vi "subbocht.vi"(4 "tijdsinterval 6":dbl, 5 "Boolean":bool, 6 "tijdsinterval 8":dbl, 7 "tijdsinterval in":dbl, 8 "tijdsinterval 7":dbl, 9 "tijdsinterval 5":dbl, 10 "tijdsinterval 4":dbl, 11 "tijdsinterval 3":dbl) -> ()   [LabVIEW 2019]
uses:
  Global 1.vi
  <vilib>/myRIO/Common/Instrument Driver Framework/Utilities/typedefs/Analog Scaling Constants.ctl
  <vilib>/myRIO/Common/Instrument Driver Framework/Utilities/typedefs/Analog Scaling Constants List.ctl
  <vilib>/myRIO/Common/Instrument Driver Framework/myRIO v1.0/AO/typedefs/AO Channels Enum.ctl
  <vilib>/myRIO/Common/Instrument Driver Framework/myRIO v1.0/AO/typedefs/AO Channels List.ctl
  <vilib>/myRIO/Common/Instrument Driver Framework/Utilities/typedefs/Generic FPGA Reference.ctl
  <vilib>/myRIO/Common/Instrument Driver Framework/Utilities/typedefs/myRIO v1.0 Reference.ctl
  <vilib>/myRIO/Common/Instrument Driver Framework/Utilities/typedefs/Hardware Version Enum.ctl
  <vilib>/myRIO/Common/Instrument Driver Framework/Utilities/typedefs/myRIO Generic Hardware Reference.ctl
  <vilib>/myRIO/Instrument Drivers/Onboard IO/AO/typedefs/AO Reference.ctl
  <vilib>/myRIO/Instrument Drivers/Onboard IO/AO/AO.lvlib
  <vilib>/myRIO/Instrument Drivers/Onboard IO/AO/vis/Write.vi
  <vilib>/userDefined/High Color/nirio_resource_hc.ctl
  <vilib>/myRIO/Common/Instrument Driver Framework/myRIO v1.0/AO/vis/myRIO v1.1 Open AO.vi
  <vilib>/myRIO/Instrument Drivers/Onboard IO/AO/vis/myRIO AO Open.xnode
  <vilib>/myRIO/Common/Instrument Driver Framework/Utilities/vis/Is FPGA Ref Available.vi
  <vilib>/myRIO/Express VI/Onboard IO/AO/AO Express VI.xnode
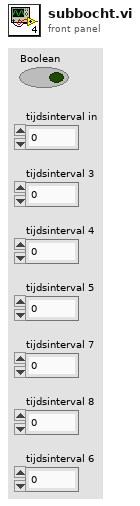
[diagram p1: front panel]
types:
  T1 = typedef "AO.lvlib/AO Reference.ctl" = cluster{"myRIO Reference":T2, "AO Channel List":T6, "AO Scaling Constant List":T8}
  T2 = typedef "myRIO Generic Hardware Reference.ctl" = cluster{"myRIO Model":T3, "myRIO Hardware Reference":T4}
  T3 = typedef "Hardware Version Enum.ctl" = enum16{"Unknown", "myRIO-1900", "myRIO-1950", "roboRIO", "NI ELVIS RIO CM", "ELVIS III"}
  T4 = typedef "myRIO v1.0 Reference.ctl" = cluster{"Generic FPGA Reference":T5, "Allow multiple opens":bool}
  T5 = typedef "Generic FPGA Reference.ctl" = refnum<k20>
  T6 = typedef "AO Channels List.ctl" = T7[]
  T7 = typedef "AO Channels Enum.ctl" = enum16{"Not Connected", "AudioOut/Left", "AudioOut/Right", "C/AO0", "C/AO1", "A/AO0", "A/AO1", "B/AO0", "B/AO1"}
  T8 = typedef "Analog Scaling Constants List.ctl" = T9[]
  T9 = typedef "Analog Scaling Constants.ctl" = cluster{"LSB Weight (Volts)":dbl, "Offset (Volts)":dbl, "Signed?":bool}
  T10 = typedef "nirio_resource_hc.ctl" = tag
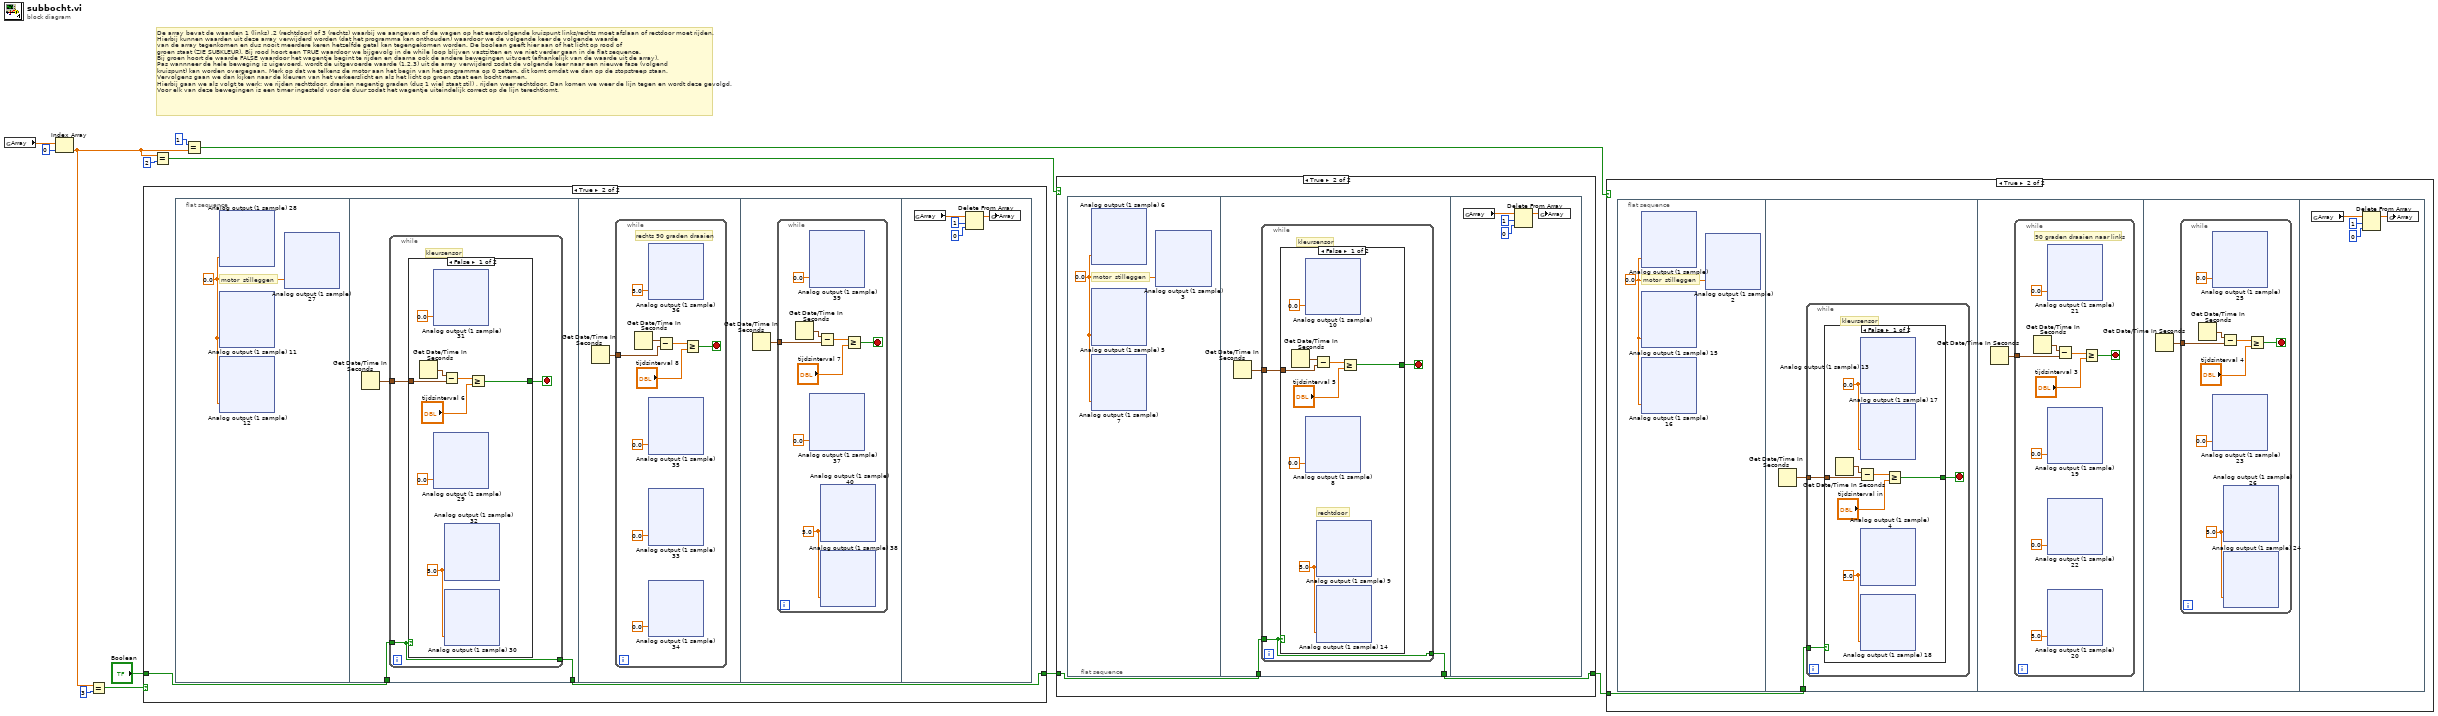
[diagram p0: block diagram]
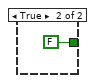
[diagram p3: hidden frame]
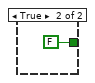
[diagram p5: hidden frame]
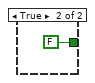
[diagram p7: hidden frame]
diagram:
  # "De array bevat de waarden 1 (links) ,2 (rechtdoor) of 3 (rechts) waarbij we aangeven of de wagen op het eerstvolgende kruispunt links/rechts moet afslaan of rectdoor moet rijden.\nHierbij kunnen waarden uit deze array verwijderd worden (dat het programma kan onthouden) waardoor we de volgende keer de volgende waarde \nvan de array tegenkomen en dus nooit meerdere keren hetzelfde getal kan tegengekomen worden. De boolean geeft hier aan of het licht op rood of \ngroen staat (ZIE SUBKLEUR). Bij rood hoort een TRUE waardoor we bijgevolg in de while loop blijven vastzitten en we niet verder gaan in de flat sequence.\nBij groen hoort de waarde FALSE waardoor het wagentje begint te rijden en daarna ook de andere bewegingen uitvoert (afhankelijk van de waarde uit de array).\nPas wannneer de hele beweging is uigevoerd, wordt de uitgevoerde waarde (1,2,3) uit de array verwijderd zodat de volgende keer naar een nieuwe fase (volgend\nkruispunt) kan worden overgegaan. Merk op dat we telkens de motor aan het begin van het programma op 0 zetten, dit komt omdat we dan op de stopstreep staan.\nVervolgens gaan we dan kijken naar de kleuren van het verkeerslicht en als het licht op groen staat een bocht nemen.\nHierbij gaan we als volgt te werk: we rijden rechttdoor, draaien negentig graden (dus 1 wiel staat stil) , rijden weer rechtdoor. Dan komen we weer de lijn tegen en wordt deze gevolgd.\nVoor elk van deze bewegingen is een timer ingesteld voor de duur zodat het wagentje uiteindelijk correct op de lijn terechtkomt."
  n1 = global read "Global 1.vi" "Array"() -> (w4:dbl[])
  n2 = Index Array(array=w4, index=0) -> (element=w6:dbl)
  n3 = Equal?(x=w6, y=3) -> (x = y?=w3:bool)
  n4 = case shown="True" w3 {
    tunnel: "Boolean" -> [w13 w15]
    tunnel: [w13 w14] -> w11
    frame False {
    }
    frame True {
      n5 = flat-sequence {
        tunnel: w15 -> [w167]
        tunnel: [w166] -> w14
        frame #0 {
          w16 = 0.0
          # "motor  stilleggen"
          n6 = xnode "Analog output (1 sample) 28"("A/AO1 (Pin 4)"=w16) -> ()  [unwired: 1 in, 1 out]
          n7 = xnode "Analog output (1 sample) 11"("B/AO0 (Pin 2)"=w16) -> ()  [unwired: 1 in, 1 out]
          n8 = xnode "Analog output (1 sample) 12"("A/AO0 (Pin 2)"=w16) -> ()  [unwired: 1 in, 1 out]
          n9 = xnode "Analog output (1 sample) 27"("B/AO1 (Pin 4)"=w16) -> ()  [unwired: 1 in, 1 out]
        }
        frame #1 {
          n10 = Get Date/Time In Seconds() -> (seconds since 1Jan1904=w165:timestamp)
          n11 = while {
            tunnel: w167 -> [w169]
            tunnel: [w169] -> w166
            tunnel: w165 -> [w168]
            stop <- w170 stop-if-true
            # "kleursensor"
            n12 = case shown="False" w169 {
              tunnel: [w171 FALSE] -> w170
              tunnel: w168 -> [w172 _]
              frame False {
                w177 = 5.0
                n13 = Get Date/Time In Seconds() -> (seconds since 1Jan1904=w173:timestamp)
                n14 = xnode "Analog output (1 sample) 31"("A/AO1 (Pin 4)"=0.0) -> ()  [unwired: 1 in, 1 out]
                n15 = xnode "Analog output (1 sample) 29"("B/AO1 (Pin 4)"=0.0) -> ()  [unwired: 1 in, 1 out]
                n16 = Subtract(x=w173, y=w172) -> (x-y=w175:dbl)
                n17 = xnode "Analog output (1 sample) 32"("A/AO0 (Pin 2)"=w177) -> ()  [unwired: 1 in, 1 out]
                n18 = xnode "Analog output (1 sample) 30"("B/AO0 (Pin 2)"=w177) -> ()  [unwired: 1 in, 1 out]
                n19 = Greater Or Equal?(x=w175, y="tijdsinterval 6") -> (x >= y?=w171:bool)
              }
              frame True {
              }
            }
          }
        }
        frame #2 {
          n20 = Get Date/Time In Seconds() -> (seconds since 1Jan1904=w328:timestamp)
          n21 = while {
            tunnel: w328 -> [w330]
            stop <- w331 stop-if-true
            # "rechts 90 graden draaien"
            n22 = Get Date/Time In Seconds() -> (seconds since 1Jan1904=w334:timestamp)
            n23 = xnode "Analog output (1 sample) 36"("A/AO0 (Pin 2)"=5.0) -> ()  [unwired: 1 in, 1 out]
            n24 = xnode "Analog output (1 sample) 35"("A/AO1 (Pin 4)"=0.0) -> ()  [unwired: 1 in, 1 out]
            n25 = xnode "Analog output (1 sample) 33"("B/AO1 (Pin 4)"=0.0) -> ()  [unwired: 1 in, 1 out]
            n26 = xnode "Analog output (1 sample) 34"("B/AO0 (Pin 2)"=0.0) -> ()  [unwired: 1 in, 1 out]
            n27 = Subtract(x=w334, y=w330) -> (x-y=w332:dbl)
            n28 = Greater Or Equal?(x=w332, y="tijdsinterval 8") -> (x >= y?=w331:bool)
          }
        }
        frame #3 {
          n29 = Get Date/Time In Seconds() -> (seconds since 1Jan1904=w486:timestamp)
          n30 = while {
            tunnel: w486 -> [w488]
            stop <- w487 stop-if-true
            w493 = 5.0
            n31 = Get Date/Time In Seconds() -> (seconds since 1Jan1904=w491:timestamp)
            n32 = xnode "Analog output (1 sample) 39"("A/AO1 (Pin 4)"=0.0) -> ()  [unwired: 1 in, 1 out]
            n33 = xnode "Analog output (1 sample) 37"("B/AO1 (Pin 4)"=0.0) -> ()  [unwired: 1 in, 1 out]
            n34 = Subtract(x=w491, y=w488) -> (x-y=w489:dbl)
            n35 = xnode "Analog output (1 sample) 40"("A/AO0 (Pin 2)"=w493) -> ()  [unwired: 1 in, 1 out]
            n36 = xnode "Analog output (1 sample) 38"("B/AO0 (Pin 2)"=w493) -> ()  [unwired: 1 in, 1 out]
            n37 = Greater Or Equal?(x=w489, y="tijdsinterval 7") -> (x >= y?=w487:bool)
          }
        }
        frame #4 {
          n38 = global read "Global 1.vi" "Array"() -> (w645:dbl[])
          n39 = Delete From Array(array=w645, length=1, index=0) -> (array with subset deleted=w646:dbl[])  [unwired: 1 out]
          n40 = global write "Global 1.vi" "Array"(w646) -> ()
        }
      }
    }
  }
  n41 = Equal?(x=w6, y=2) -> (x = y?=w2:bool)
  n42 = Equal?(x=1, y=w6) -> (x = y?=w1:bool)
  n43 = case shown="True" w2 {
    tunnel: w11 -> [w647 w649]
    tunnel: [w647 w648] -> w12
    frame False {
    }
    frame True {
      n44 = flat-sequence {
        tunnel: w649 -> [w801]
        tunnel: [w800] -> w648
        frame #0 {
          w650 = 0.0
          # "motor  stilleggen"
          n45 = xnode "Analog output (1 sample) 6"("A/AO1 (Pin 4)"=w650) -> ()  [unwired: 1 in, 1 out]
          n46 = xnode "Analog output (1 sample) 5"("B/AO0 (Pin 2)"=w650) -> ()  [unwired: 1 in, 1 out]
          n47 = xnode "Analog output (1 sample) 7"("A/AO0 (Pin 2)"=w650) -> ()  [unwired: 1 in, 1 out]
          n48 = xnode "Analog output (1 sample) 3"("B/AO1 (Pin 4)"=w650) -> ()  [unwired: 1 in, 1 out]
        }
        frame #1 {
          n49 = Get Date/Time In Seconds() -> (seconds since 1Jan1904=w799:timestamp)
          n50 = while {
            tunnel: w801 -> [w803]
            tunnel: [w803] -> w800
            tunnel: w799 -> [w802]
            stop <- w804 stop-if-true
            # "kleursensor"
            n51 = case shown="False" w803 {
              tunnel: [w805 FALSE] -> w804
              tunnel: w802 -> [w806 _]
              frame False {
                w811 = 5.0
                # "rechtdoor"
                n52 = Get Date/Time In Seconds() -> (seconds since 1Jan1904=w809:timestamp)
                n53 = xnode "Analog output (1 sample) 10"("A/AO1 (Pin 4)"=0.0) -> ()  [unwired: 1 in, 1 out]
                n54 = xnode "Analog output (1 sample) 8"("B/AO1 (Pin 4)"=0.0) -> ()  [unwired: 1 in, 1 out]
                n55 = Subtract(x=w809, y=w806) -> (x-y=w807:dbl)
                n56 = xnode "Analog output (1 sample) 9"("A/AO0 (Pin 2)"=w811) -> ()  [unwired: 1 in, 1 out]
                n57 = xnode "Analog output (1 sample) 14"("B/AO0 (Pin 2)"=w811) -> ()  [unwired: 1 in, 1 out]
                n58 = Greater Or Equal?(x=w807, y="tijdsinterval 5") -> (x >= y?=w805:bool)
              }
              frame True {
              }
            }
          }
        }
        frame #2 {
          n59 = global read "Global 1.vi" "Array"() -> (w964:dbl[])
          n60 = Delete From Array(array=w964, length=1, index=0) -> (array with subset deleted=w965:dbl[])  [unwired: 1 out]
          n61 = global write "Global 1.vi" "Array"(w965) -> ()
        }
      }
    }
  }
  n62 = case shown="True" w1 {
    tunnel: w12 -> [_ w966]
    frame False {
    }
    frame True {
      n63 = flat-sequence {
        tunnel: w966 -> [w1117]
        frame #0 {
          w967 = 0.0
          # "motor  stilleggen"
          n64 = xnode "Analog output (1 sample)"("A/AO1 (Pin 4)"=w967) -> ()  [unwired: 1 in, 1 out]
          n65 = xnode "Analog output (1 sample) 15"("B/AO1 (Pin 4)"=w967) -> ()  [unwired: 1 in, 1 out]
          n66 = xnode "Analog output (1 sample) 16"("A/AO0 (Pin 2)"=w967) -> ()  [unwired: 1 in, 1 out]
          n67 = xnode "Analog output (1 sample) 2"("B/AO0 (Pin 2)"=w967) -> ()  [unwired: 1 in, 1 out]
        }
        frame #1 {
          n68 = Get Date/Time In Seconds() -> (seconds since 1Jan1904=w1116:timestamp)
          n69 = while {
            tunnel: w1117 -> [w1119]
            tunnel: w1116 -> [w1118]
            stop <- w1120 stop-if-true
            # "kleursensor"
            n70 = case shown="False" w1119 {
              tunnel: [w1122 FALSE] -> w1120
              tunnel: w1118 -> [w1121 _]
              frame False {
                w1126 = 0.0
                w1127 = 5.0
                n71 = Get Date/Time In Seconds() -> (seconds since 1Jan1904=w1125:timestamp)
                n72 = Subtract(x=w1125, y=w1121) -> (x-y=w1123:dbl)
                n73 = xnode "Analog output (1 sample) 13"("A/AO1 (Pin 4)"=w1126) -> ()  [unwired: 1 in, 1 out]
                n74 = xnode "Analog output (1 sample) 17"("B/AO1 (Pin 4)"=w1126) -> ()  [unwired: 1 in, 1 out]
                n75 = xnode "Analog output (1 sample) 4"("A/AO0 (Pin 2)"=w1127) -> ()  [unwired: 1 in, 1 out]
                n76 = xnode "Analog output (1 sample) 18"("B/AO0 (Pin 2)"=w1127) -> ()  [unwired: 1 in, 1 out]
                n77 = Greater Or Equal?(x=w1123, y="tijdsinterval in") -> (x >= y?=w1122:bool)
              }
              frame True {
              }
            }
          }
        }
        frame #2 {
          n78 = Get Date/Time In Seconds() -> (seconds since 1Jan1904=w1277:timestamp)
          n79 = while {
            tunnel: w1277 -> [w1280]
            stop <- w1279 stop-if-true
            # "90 graden draaien naar links"
            n80 = Get Date/Time In Seconds() -> (seconds since 1Jan1904=w1283:timestamp)
            n81 = xnode "Analog output (1 sample) 21"("A/AO1 (Pin 4)"=0.0) -> ()  [unwired: 1 in, 1 out]
            n82 = xnode "Analog output (1 sample) 19"("B/AO1 (Pin 4)"=0.0) -> ()  [unwired: 1 in, 1 out]
            n83 = xnode "Analog output (1 sample) 22"("A/AO0 (Pin 2)"=0.0) -> ()  [unwired: 1 in, 1 out]
            n84 = xnode "Analog output (1 sample) 20"("B/AO0 (Pin 2)"=5.0) -> ()  [unwired: 1 in, 1 out]
            n85 = Subtract(x=w1283, y=w1280) -> (x-y=w1281:dbl)
            n86 = Greater Or Equal?(x=w1281, y="tijdsinterval 3") -> (x >= y?=w1279:bool)
          }
        }
        frame #3 {
          n87 = Get Date/Time In Seconds() -> (seconds since 1Jan1904=w1435:timestamp)
          n88 = while {
            tunnel: w1435 -> [w1437]
            stop <- w1436 stop-if-true
            w1442 = 5.0
            n89 = Get Date/Time In Seconds() -> (seconds since 1Jan1904=w1440:timestamp)
            n90 = xnode "Analog output (1 sample) 25"("A/AO1 (Pin 4)"=0.0) -> ()  [unwired: 1 in, 1 out]
            n91 = xnode "Analog output (1 sample) 23"("B/AO1 (Pin 4)"=0.0) -> ()  [unwired: 1 in, 1 out]
            n92 = Subtract(x=w1440, y=w1437) -> (x-y=w1438:dbl)
            n93 = xnode "Analog output (1 sample) 26"("A/AO0 (Pin 2)"=w1442) -> ()  [unwired: 1 in, 1 out]
            n94 = xnode "Analog output (1 sample) 24"("B/AO0 (Pin 2)"=w1442) -> ()  [unwired: 1 in, 1 out]
            n95 = Greater Or Equal?(x=w1438, y="tijdsinterval 4") -> (x >= y?=w1436:bool)
          }
        }
        frame #4 {
          n96 = global read "Global 1.vi" "Array"() -> (w1595:dbl[])
          n97 = Delete From Array(array=w1595, length=1, index=0) -> (array with subset deleted=w1594:dbl[])  [unwired: 1 out]
          n98 = global write "Global 1.vi" "Array"(w1594) -> ()
        }
      }
    }
  }
